vi "sv_Check Data Valid (Audio) (1 Ch).vi"(0 "complex spectrum":T8={"complex spectrum response"={"f0"=0.0, "df"=1.0, "complex spectrum"=[]}, "spectrum info"={"channel name"="", "description"="", "x-axis units"=0, "spectral info"={"spectrum type"=enum."Power [Magnitude^2]", "linear/dB"=enum."linear", "window"=0, "window size"=0, "FFT size"=0}, "engineering units"=0, "custom label"="", "dB reference [EU]"=0.0, "peak units"=enum."rms", "weighting filter"=0, "spectral density?"=FALSE, "unit label"="", "spectrum skewed?"=FALSE, "complimentary spectrum units"=enum."none"}} {"spectrum info"."x-axis units" items=["Time (s)"=0, "Frequency-CB (Hz)"=1, "Frequency-CPB (Hz)"=1248, "Frequency-Arbitrary (Hz)"=2357, "Quefrency (s)"=2, "Revolutions (rev)"=3, "Order"=4, "Speed (RPM)"=11, "Speed (rad/s)"=21, "Index"=65535]; "spectrum info"."weighting filter" items=["Linear", "A-weighting", "B-weighting", "C-weighting", "ITU-R 468-4", "Dolby", "CCITT", "C-message", "Wb", "Wc", "Wd", "We", "Wf", "Wh", "Wj", "Wk", "Wm", "AES17 20 kHz lowpass", "AES17 40 kHz lowpass", "AES17 20 kHz highpass", "AES17 40 kHz highpass"]; "spectrum info"."dB reference [EU]" format="%.2f"; "spectrum info"."engineering units" items=["custom..."=0, "V"=1, "A"=21, "C"=30, "pC"=31, "s"=32, "-"=29, "Pa"=2, "N"=20, "g"=3, "m/s^2"=4, "m/s"=5, "m"=6, "mm/s"=12, "mm"=13, "micron/s"=14, "micron"=15, "in/s^2"=7, "in/s"=8, "in"=9, "mil/s"=10, "mil"=11, "rad/s^2"=16, "rad/s"=17, "rad"=18, "deg/s^2"=26, "deg/s"=27, "deg"=28, "RPM"=22, "cycle/s^2"=23, "Hz"=24, "cycle"=25, "strain"=19]; "spectrum info"."spectral info"."window" items=["None "=0, "Hanning"=1, "Hamming"=2, "Blackman-Harris"=3, "Exact Blackman"=4, "Blackman"=5, "Flat Top"=6, "4 Term B-Harris "=7, "7 Term B-Harris"=8, "Low Sidelobe"=9, "Force - Exponential"=10, "Gaussian"=62]; "complex spectrum response"."complex spectrum" format="%.2f"; "complex spectrum response"."df" format="%.2f"; "complex spectrum response"."f0" format="%.2f"}, 1 "IMD standard":T1(ring)=enum."Custom", 2 "custom IMD signal":T9={"IMD type"=enum."SMPTE/DIN", "low-frequency tone"=-1.0, "high-frequency tone"=-1.0, "amplitude ratio"=-1.0, "maximum order"=-1} {"amplitude ratio" format="%.1f"; "high-frequency tone" format="%.2f"; "low-frequency tone" format="%.2f"}, 3 "frequency range in":T10={"start frequency"=-1.0, "stop frequency"=-1.0} {"stop frequency" format="%.2f"; "start frequency" format="%.2f"}, 5 "error in (no error)":errorcluster, 6 "harmonics to visualize":i32[](array[numeric]), 7 "amplitude":dbl=-1.0 format="%.3f", 8 "maximum harmonic":i32, 9 "expected fundamental frequency [Hz]":dbl=-1.0 format="%.2f") -> (10 "dup maximum harmonic":i32=2, 11 "dup expected fundamental frequency [Hz]":dbl=-1.0 format="%.2f", 12 "dup harmonics to visualize":i32[](array[numeric])=[2], 13 "dup amplitude":dbl format="%.2f", 14 "complex spectrum":T8={"complex spectrum response"={"f0"=0.0, "df"=1.0, "complex spectrum"=[]}, "spectrum info"={"channel name"="", "description"="", "x-axis units"=0, "spectral info"={"spectrum type"=enum."Power [Magnitude^2]", "linear/dB"=enum."linear", "window"=0, "window size"=0, "FFT size"=0}, "engineering units"=0, "custom label"="", "dB reference [EU]"=0.0, "peak units"=enum."rms", "weighting filter"=0, "spectral density?"=FALSE, "unit label"="", "spectrum skewed?"=FALSE, "complimentary spectrum units"=enum."none"}} {"spectrum info"."x-axis units" items=["Time (s)"=0, "Frequency-CB (Hz)"=1, "Frequency-CPB (Hz)"=1248, "Frequency-Arbitrary (Hz)"=2357, "Quefrency (s)"=2, "Revolutions (rev)"=3, "Order"=4, "Speed (RPM)"=11, "Speed (rad/s)"=21, "Index"=65535]; "spectrum info"."weighting filter" items=["Linear", "A-weighting", "B-weighting", "C-weighting", "ITU-R 468-4", "Dolby", "CCITT", "C-message", "Wb", "Wc", "Wd", "We", "Wf", "Wh", "Wj", "Wk", "Wm", "AES17 20 kHz lowpass", "AES17 40 kHz lowpass", "AES17 20 kHz highpass", "AES17 40 kHz highpass"]; "spectrum info"."dB reference [EU]" format="%.2f"; "spectrum info"."engineering units" items=["custom..."=0, "V"=1, "A"=21, "C"=30, "pC"=31, "s"=32, "-"=29, "Pa"=2, "N"=20, "g"=3, "m/s^2"=4, "m/s"=5, "m"=6, "mm/s"=12, "mm"=13, "micron/s"=14, "micron"=15, "in/s^2"=7, "in/s"=8, "in"=9, "mil/s"=10, "mil"=11, "rad/s^2"=16, "rad/s"=17, "rad"=18, "deg/s^2"=26, "deg/s"=27, "deg"=28, "RPM"=22, "cycle/s^2"=23, "Hz"=24, "cycle"=25, "strain"=19]; "spectrum info"."spectral info"."window" items=["None "=0, "Hanning"=1, "Hamming"=2, "Blackman-Harris"=3, "Exact Blackman"=4, "Blackman"=5, "Flat Top"=6, "4 Term B-Harris "=7, "7 Term B-Harris"=8, "Low Sidelobe"=9, "Force - Exponential"=10, "Gaussian"=62]; "complex spectrum response"."complex spectrum" format="%.2f"; "complex spectrum response"."df" format="%.2f"; "complex spectrum response"."f0" format="%.2f"}, 16 "dup custom IMD signal":T9={"IMD type"=enum."CCIF/Twin-Tone", "low-frequency tone"=14000.0, "high-frequency tone"=15000.0, "amplitude ratio"=1.0, "maximum order"=5} {"amplitude ratio" format="%.1f"; "high-frequency tone" format="%.2f"; "low-frequency tone" format="%.2f"}, 17 "frequency range out":T10={"start frequency"=0.0, "stop frequency"=499.0} {"stop frequency" format="%.2f"; "start frequency" format="%.2f"}, 19 "error out":errorcluster)   [LabVIEW 2017, in "SoundVib_Distortion.lvlib"]
uses:
  <vilib>/addons/Sound and Vibration/svt_Distortion/SoundVib_Distortion.lvlib
  <vilib>/addons/_NISVFA/_Shared subVIs/Controls/svc_Spectrum Info.ctl
  <vilib>/addons/_NISVFA/_Shared subVIs/Controls/svc_X-Axis Units.ctl
  <vilib>/addons/_NISVFA/_Shared subVIs/Controls/svc_Spectrum Type.ctl
  <vilib>/addons/_NISVFA/_Shared subVIs/Controls/svc_Engineering Units Text Ring.ctl
  <vilib>/addons/_NISVFA/_Shared subVIs/Controls/svc_Weighting Filter Text Ring.ctl
  <vilib>/addons/_NISVFA/_Shared subVIs/Controls/svc_Complimentary Spectrum Units.ctl
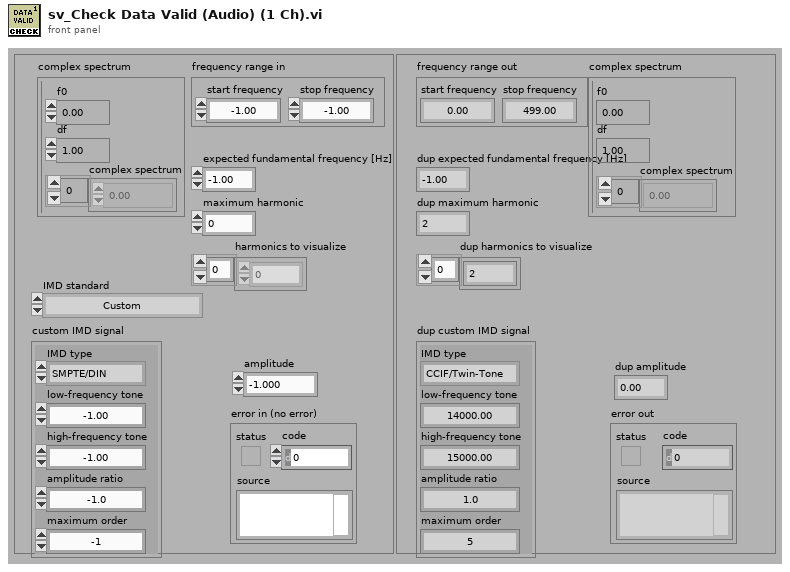
[diagram p1: front panel]
types:
  T1 = enum16{"SMPTE (60 Hz, 7000 Hz, 4:1)", "DIN (250 Hz, 8000 Hz, 4:1)", "CCIF (11 kHz, 12 kHz, 1:1)", "CCIF (19 kHz, 20 kHz, 1:1)", "Custom"}
  T2 = typedef "svc_Spectrum Info.ctl" = cluster{"channel name":string, "description":string, "x-axis units":T3, "spectral info":cluster{"spectrum type":T4, "linear/dB":enum16{"linear", "dB"}, "window":u16, "window size":i32, "FFT size":i32}, "engineering units":T5, "custom label":string, "dB reference [EU]":dbl, "peak units":enum16{"rms", "peak", "peak-peak"}, "weighting filter":T6, "spectral density?":bool, "unit label":string, "spectrum skewed?":bool, "complimentary spectrum units":T7}
  T3 = typedef "svc_X-Axis Units.ctl" = u16
  T4 = typedef "svc_Spectrum Type.ctl" = enum16{"FFT Spectrum [complex]", "Amplitude [Magnitude]", "Power [Magnitude^2]", "Cross Spectrum [complex]", "Frequency Response [Complex]"}
  T5 = typedef "svc_Engineering Units Text Ring.ctl" = u16
  T6 = typedef "svc_Weighting Filter Text Ring.ctl" = u16
  T7 = typedef "svc_Complimentary Spectrum Units.ctl" = enum16{"none", "radians", "degrees", "cycles", "imaginary"}
  T8 = cluster{"complex spectrum response":cluster{"f0":dbl, "df":dbl, "complex spectrum":cdb[]}, "spectrum info":T2}
  T9 = cluster{"IMD type":enum16{"SMPTE/DIN", "CCIF/Twin-Tone"}, "low-frequency tone":dbl, "high-frequency tone":dbl, "amplitude ratio":dbl, "maximum order":i32}
  T10 = cluster{"start frequency":dbl, "stop frequency":dbl}
  T11 = enum16{"FFT Spectrum [complex]", "Amplitude [Magnitude]", "Power [Magnitude^2]", "Cross Spectrum [complex]", "Frequency Response [Complex]"}
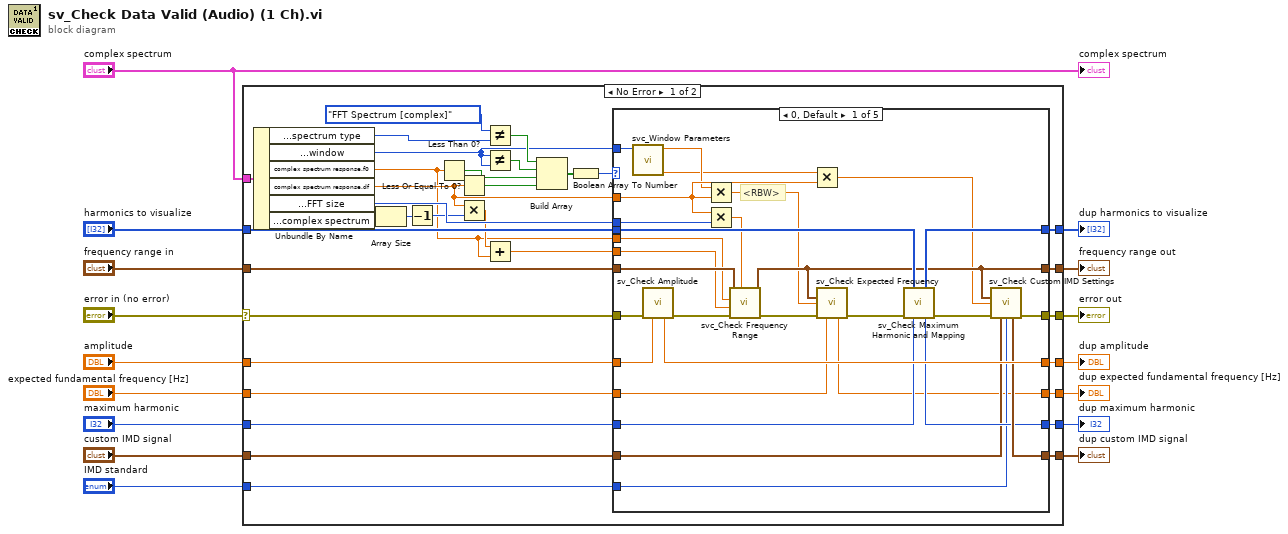
[diagram p0: block diagram]
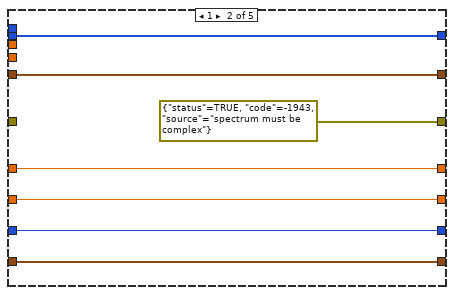
[diagram p2: hidden frame]
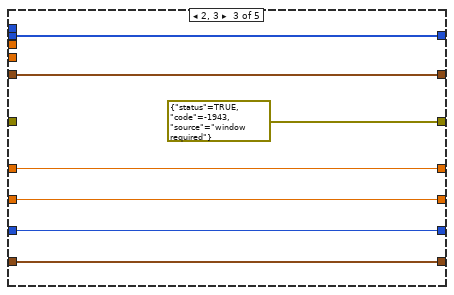
[diagram p3: hidden frame]
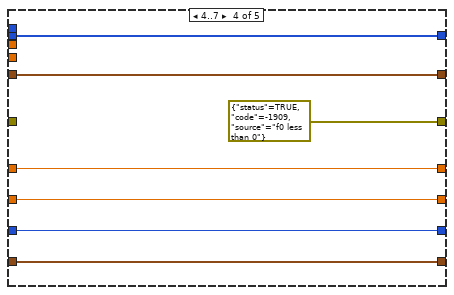
[diagram p4: hidden frame]
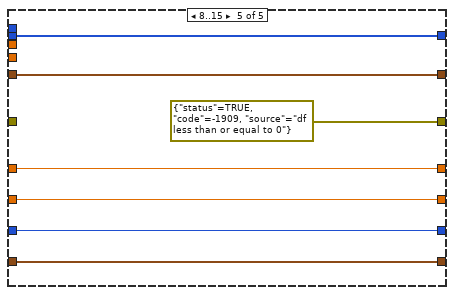
[diagram p5: hidden frame]
diagram:
  n1 = case shown="No Error" "error in (no error)" {
    selector: "error in (no error)" -> [w45 w113]
    tunnel: "frequency range in" -> [w37 w112]
    tunnel: [w36 w112] -> w15
    tunnel: "expected fundamental frequency [Hz]" -> [w44 w108]
    tunnel: [w47 w113] -> w12
    tunnel: "maximum harmonic" -> [w43 w110]
    tunnel: "amplitude" -> [w49 w109]
    tunnel: "custom IMD signal" -> [w41 w107]
    tunnel: [w42 w110] -> w6
    tunnel: [w48 w109] -> w5
    tunnel: [w40 w108] -> w4
    tunnel: [w46 w107] -> w3
    tunnel: "harmonics to visualize" -> [w38 w111]
    tunnel: [w39 w111] -> w10
    tunnel: "complex spectrum" -> [w31 _]
    tunnel: "IMD standard" -> [w34 _]
    frame No Error {
      n2 = Unbundle By Name(w31) -> ("spectrum info.spectral info.spectrum type"=w35:T4, "spectrum info.spectral info.window"=w24:u16, "complex spectrum response.f0"=w18:dbl, "complex spectrum response.df"=w20:dbl, "spectrum info.spectral info.FFT size"=w25:i32, "complex spectrum response.complex spectrum"=w23:cdb[])
      n3 = Array Size(array=w23) -> (size(s)=w22:i32)
      n4 = Decrement(x=w22) -> (x-1=w21:i32)
      n5 = Less Than 0?(x=w18) -> (x < 0?=w29:bool)
      n6 = Less Or Equal To 0?(x=w20) -> (x <= 0?=w30:bool)
      n7 = Multiply(x=w20, y=w21) -> (x*y=w19:dbl)
      n8 = Not Equal?(x=T11."FFT Spectrum [complex]", y=w35) -> (x != y?=w26:bool)
      n9 = Not Equal?(x=w24, y=w24) -> (x != y?=w27:bool)
      n10 = Add(x=w19, y=w18) -> (x+y=w17:dbl)
      n11 = Build Array(w26, w27, w29, w30) -> (w33:bool[])
      n12 = Boolean Array To Number(Boolean array=w33) -> (number=w32:u32)
      n13 = case shown="0, Default" w32 {
        tunnel: w49 -> [w77 w84 w89 w97 w104]
        tunnel: [w76 w84 w89 w97 w104] -> w48
        tunnel: [w75 errorcluster {"status"=TRUE, "code"=-1943, "source"="spectrum must be complex"} ("error IO") errorcluster {"status"=TRUE, "code"=-1943, "source"="window required"} ("error IO") errorcluster {"status"=TRUE, "code"=-1909, "source"="f0 less than 0"} ("error IO") errorcluster {"status"=TRUE, "code"=-1909, "source"="df less than or equal to 0"} ("error IO")] -> w47
        tunnel: [w74 w81 w86 w94 w101] -> w46
        tunnel: w45 -> [w73 _ _ _ _]
        tunnel: w44 -> [w71 w83 w88 w96 w103]
        tunnel: w43 -> [w69 w82 w87 w95 w102]
        tunnel: [w68 w82 w87 w95 w102] -> w42
        tunnel: w41 -> [w65 w81 w86 w94 w101]
        tunnel: [w57 w83 w88 w96 w103] -> w40
        tunnel: [w64 w80 w91 w99 w106] -> w39
        tunnel: w38 -> [w63 w80 w91 w99 w106]
        tunnel: w37 -> [w62 w85 w90 w98 w105]
        tunnel: [w59 w85 w90 w98 w105] -> w36
        tunnel: w25 -> [w52 _ _ _ _]
        tunnel: w34 -> [w60 _ _ _ _]
        tunnel: w20 -> [w78 _ _ _ _]
        tunnel: w24 -> [w56 _ _ _ _]
        tunnel: w18 -> [w53 _ _ _ _]
        tunnel: w17 -> [w51 _ _ _ _]
        frame 0, Default {
          # "<RBW>"
          n14 = call <vilib>:"svc_Window Parameters.vi"("window"=w56) -> ("maximum BW"=w50:dbl, "ENBW"=w55:dbl)  [unwired: 7 in, 2 out]
          n15 = call <vilib>:"sv_Check Amplitude.vi"("error in (no error)"=w73, "amplitude"=w77) -> ("dup amplitude"=w76:dbl, "error out"=w72:errorcluster)  [unwired: 12 in]
          n16 = Multiply(x=w55, y=w78) -> (x*y=w58:dbl)
          n17 = Multiply(x=w78, y=w52) -> (x*y=w61:dbl)
          n18 = call <vilib>:"svc_Check Frequency Range.vi"("fs"=w61, "error in (no error)"=w72, "fmax"=w51, "f0"=w53, "frequency range in"=w62) -> ("error out"=w70:errorcluster, "frequency range out"=w59:T10)  [unwired: 4 in, 1 out]
          n19 = Multiply(x=w50, y=w78) -> (x*y=w54:dbl)
          n20 = call <vilib>:"sv_Check Expected Frequency.vi"("frequency range"=w59, "RBW"=w58, "error in (no error)"=w70, "expected fundamental frequency [Hz]"=w71) -> ("dup expected fundamental frequency [Hz]"=w57:dbl, "error out"=w67:errorcluster)  [unwired: 10 in]
          n21 = call <vilib>:"sv_Check Maximum Harmonic and Mapping.vi"("harmonics to visualize in"=w63, "error in (no error)"=w67, "maximum harmonic in"=w69) -> ("dup harmonics to visualize"=w64:i32[], "dup maximum harmonic"=w68:i32, "error out"=w66:errorcluster)  [unwired: 10 in]
          n22 = call <vilib>:"sv_Check Custom IMD Settings.vi"("frequency range"=w59, "RBW"=w54, "error in (no error)"=w66, "custom IMD settings"=w65, "IMD standard"=w60) -> ("dup custom IMD settings"=w74:T9, "error out"=w75:errorcluster)  [unwired: 9 in]
        }
        frame 1 {
        }
        frame 2, 3 {
        }
        frame 4..7 {
        }
        frame 8..15 {
        }
      }
    }
    frame Error {
    }
  }
  "error out" <- w12
  "frequency range out" <- w15
  "dup harmonics to visualize" <- w10
  "dup maximum harmonic" <- w6
  "dup amplitude" <- w5
  "dup expected fundamental frequency [Hz]" <- w4
  "dup custom IMD signal" <- w3
  "complex spectrum" <- "complex spectrum"
